vi "Acquire.vi"(8 "error in (no error)":errorcluster, 11 "HW Refnum In":string) -> (0 "error out":errorcluster, 2 "Graph Data":waveform(dbl)[](array[waveform]), 3 "HW Refnum Out":string)   [LabVIEW 2020, in "Acquisition.lvlib"]
doc: "Perform the acquisition. Replace the contents of this diagram with calls to acquisition hardware.\n_____\nBased on DQMH Project Template 6.0.0.91."
uses:
  Acquisition.lvlib
  <vilib>/DAQmx/read.llb/DAQmx Read (Analog 1D Wfm NChan NSamp).vi
  <vilib>/DAQmx/miscellaneous.llb/DAQmx Fill In Error Info.vi
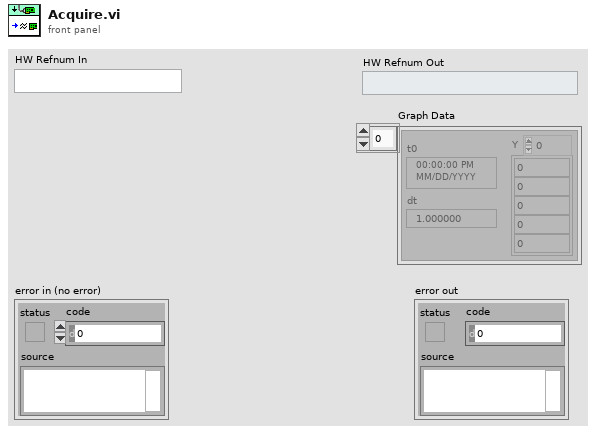
[diagram p1: front panel]
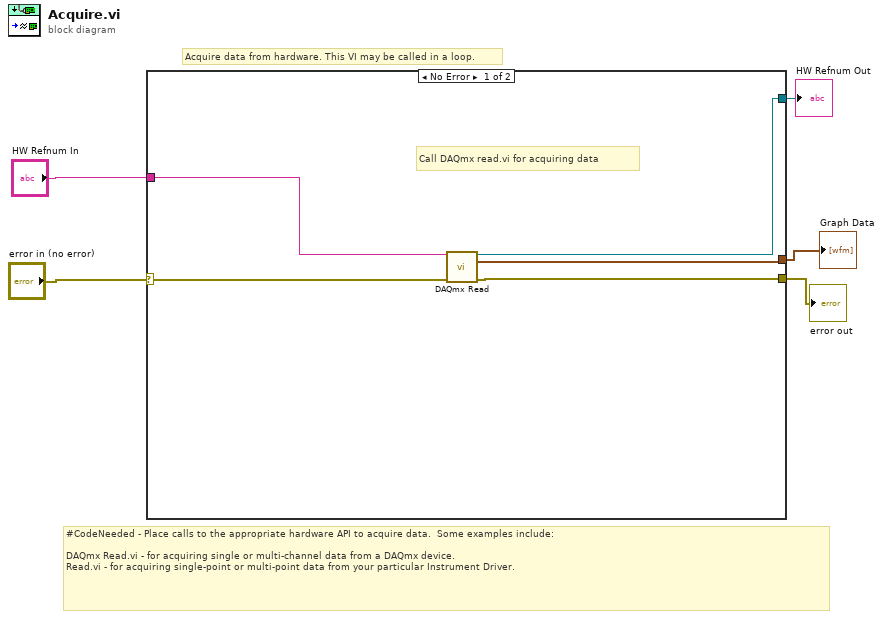
[diagram p0: block diagram]
diagram:
  # "Acquire data from hardware. This VI may be called in a loop."
  # "#CodeNeeded - Place calls to the appropriate hardware API to acquire data.  Some examples include:\n\nDAQmx Read.vi - for acquiring single or multi-channel data from a DAQmx device.\nRead.vi - for acquiring single-point or multi-point data from your particular Instrument Driver."
  n1 = case shown="No Error" "error in (no error)" {
    selector: "error in (no error)" -> [w8 w12]
    tunnel: [w7 w12] -> w4
    tunnel: [w10 w11] -> w1
    tunnel: [w9 _] -> w3
    tunnel: "HW Refnum In" -> [w6 w11]
    frame No Error {
      # "Call DAQmx read.vi for acquiring data"
      n2 = call-poly <vilib>:"DAQmx Read.vi"("task/channels in"=w6, "error in"=w8) -> ("task out"=w10:refnum<k21>, "data"=w9:waveform(dbl)[], "error out"=w7:errorcluster)  [unwired: 11 in]
    }
    frame Error {
    }
  }
  "error out" <- w4
  "Graph Data" <- w3
  "HW Refnum Out" <- w1
